vi "Labview_Test.vi"() -> ()   [LabVIEW 2011]
panel:
  out "Numeric 2":dbl
  out "Numeric":dbl
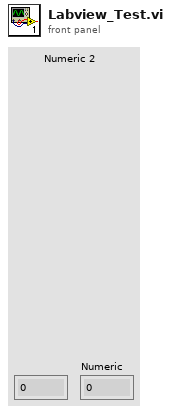
[diagram p1: front panel]
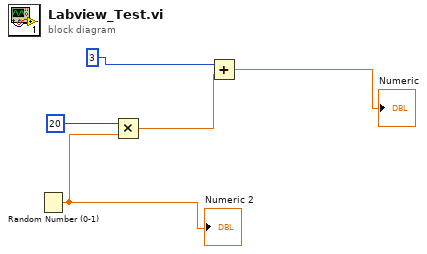
[diagram p0: block diagram]
diagram:
  n1 = Random Number (0-1)() -> (number: 0 to 1=w1:dbl)
  "Numeric 2" <- w1
  n2 = Multiply(x=20, y=w1) -> (x*y=w5:dbl)
  n3 = Add(x=3, y=w5) -> (x+y=→"Numeric":dbl)
